vi "Follow Redirects.vi"(8 "error in (no error)":errorcluster, 9 "Body":string, 10 "Headers":string, 11 "client handle":T1) -> (0 "error out":errorcluster, 1 "Body from final location":string, 2 "Headers from final location":string, 3 "client handle out":T1, 4 "response code from final location":i32)   [LabVIEW 2012]
uses:
  <vilib>/httpClient/ClientHandle.ctl
  <vilib>/httpClient/LabVIEWHTTPClient.lvlib
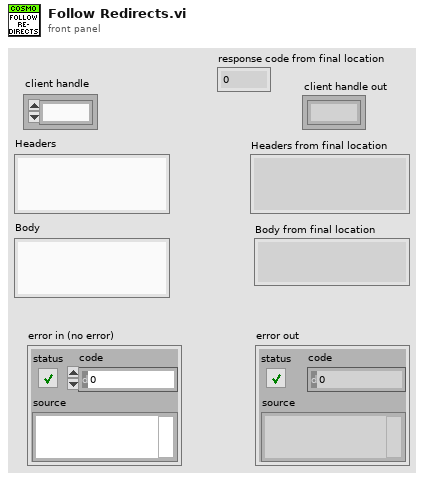
[diagram p1: front panel]
types:
  T1 = typedef "LabVIEWHTTPClient.lvlib/ClientHandle.ctl" = refnum<k1>
  T2 = typedef "Key-Value Pair.ctl" = cluster{"Key":string, "Value":string}
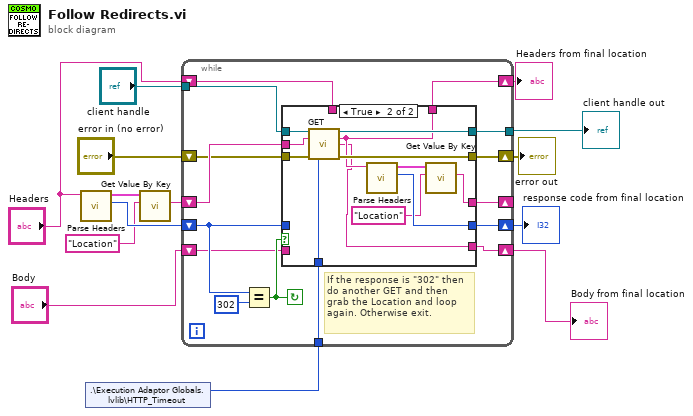
[diagram p0: block diagram]
diagram:
  n1 = call "Parse Headers.vi"("Raw Header"="Headers") -> ("response code"=w10:i32, "Parsed Headers"=w8:T2[])  [unwired: 9 in]
  n2 = shared-variable ".\\Execution Adaptor Globals.lvlib\\HTTP_Timeout"() -> (w1:i32)  [unwired: 1 in, 1 out]
  n3 = call "Get Value By Key.vi"("Key"="Location", "Key-Value Pairs"=w8) -> ("Value"=w7:string)  [unwired: 9 in]
  n4 = while {
    tunnel: "client handle" -> [w29]
    shift-right: [w27] -> w2
    shift-left: w10 -> [w26]
    shift-right: [w23] -> _
    shift-left: w7 -> [w24]
    shift-right: [w21] -> w12
    shift-left: "error in (no error)" -> [w22]
    tunnel: [w20] -> w11
    shift-right: [w18] -> w5
    shift-left: "Headers" -> [w19]
    shift-right: [w16] -> w3
    shift-left: "Body" -> [w17]
    tunnel: w1 -> [w15]
    stop <- w25 continue-if-true
    # "If the response is \"302\" then\ndo another GET and then\ngrab the Location and loop \nagain. Otherwise exit."
    n5 = Equal?(x=w26, y=302) -> (x = y?=w25:bool)
    n6 = case shown="True" w25 {
      tunnel: w29 -> [w32 w47]
      tunnel: [w35 w46] -> w27
      tunnel: w26 -> [w35 _]
      tunnel: w24 -> [w34 w45]
      tunnel: [w34 w42] -> w23
      tunnel: w22 -> [w33 w41]
      tunnel: [w33 w40] -> w21
      tunnel: [w32 w39] -> w20
      tunnel: w19 -> [w31 _]
      tunnel: [w31 w38] -> w18
      tunnel: w17 -> [w30 _]
      tunnel: [w30 w37] -> w16
      tunnel: w15 -> [_ w36]
      frame False {
      }
      frame True {
        n7 = call <vilib>:"GET.vi"("client handle"=w47, "url"=w45, "error in (no error)"=w41, "timeout (10000)"=w36) -> ("client handle out"=w39:T1, "headers"=w38:string, "body"=w37:string, "error out"=w40:errorcluster)  [unwired: 8 in]
        n8 = call "Parse Headers.vi"("Raw Header"=w38) -> ("response code"=w46:i32, "Parsed Headers"=w44:T2[])  [unwired: 9 in]
        n9 = call "Get Value By Key.vi"("Key"="Location", "Key-Value Pairs"=w44) -> ("Value"=w42:string)  [unwired: 9 in]
      }
    }
  }
  "error out" <- w12
  "client handle out" <- w11
  "Headers from final location" <- w5
  "Body from final location" <- w3
  "response code from final location" <- w2
